vi "f_to_c.vi"(8 "Fahrenheit Temperature":dbl) -> (2 "Celsius Temperature":dbl)   [LabVIEW 2021]
doc: "本VI是为《我和LabVIEW》一书编写的示例。\n关于本书的介绍请参考网页：\nhttp://ruanqizhen.spaces.live.com/blog/cns!5852D4F797C53FB6!4310.entry"
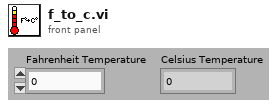
[diagram p1: front panel]
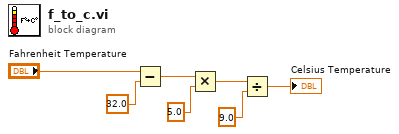
[diagram p0: block diagram]
diagram:
  n1 = Subtract(x="Fahrenheit Temperature", y=32.0) -> (x-y=w7:dbl)
  n2 = Multiply(x=w7, y=5.0) -> (x*y=w6:dbl)
  n3 = Divide(x=w6, y=9.0) -> (x/y=→"Celsius Temperature":dbl)
